vi "change_imagingMode.vi"(8 "error in (no error)":errorcluster, 10 "imagingModes":T1[](array[typedef]), 11 "imagingMode":refnum<vi>) -> (0 "error out":errorcluster)   [LabVIEW 2010]
uses:
  common/clusters/plugin_specification.ctl
  components/ImagingMode/GenericImagingMode/GenericImagingMode/GenericImagingMode.lvclass
  common/classes/GenericComponent/GenericComponent/GenericComponent.lvclass
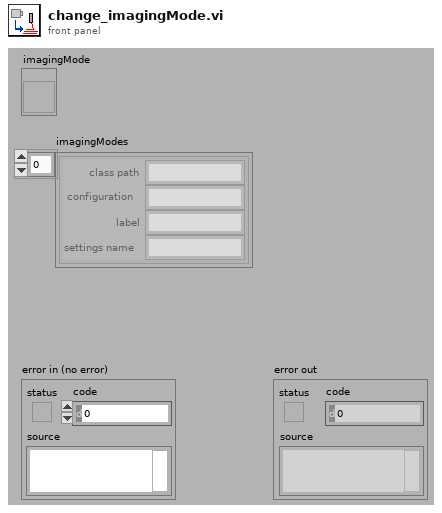
[diagram p1: front panel]
types:
  T1 = typedef "plugin_specification.ctl" = cluster{"class path":string, "configuration":string, "label":string, "settings name":string}
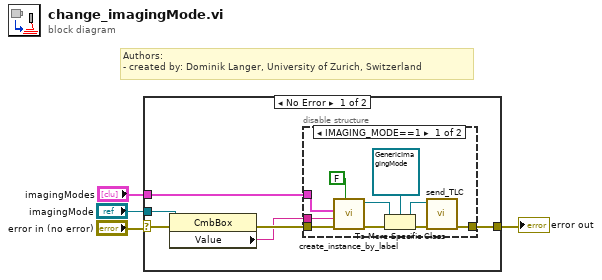
[diagram p0: block diagram]
diagram:
  # "Authors: \n- created by: Dominik Langer, University of Zurich, Switzerland"
  n1 = case shown="No Error" "error in (no error)" {
    selector: "error in (no error)" -> [w9 w22]
    tunnel: [w10 w22] -> w4
    tunnel: "imagingMode" -> [w6 _]
    tunnel: "imagingModes" -> [w5 _]
    frame No Error {
      n2 = property class="CmbBox"(reference=w6, error in=w9) -> (error out=w8:errorcluster, "Value"=w7:string)  [unwired: 1 out]
      n3 = disable-structure shown="IMAGING_MODE==1" {
        disable-tunnel: w8 -> [w16 w21]
        disable-tunnel: [w19 w21] -> w10
        disable-tunnel: w7 -> [w12 _]
        disable-tunnel: w5 -> [w11 _]
        frame condition #0 (active) {
          n4 = call "create_instance_by_label.vi"("call constructor?"=FALSE, "error in (no error)"=w16, "label"=w12, "configuration list"=w11) -> ("error out"=w15:errorcluster, "GenericPlugin out"=w14:refnum<class "GenericComponent.lvclass">)  [unwired: 6 out]
          n5 = To More Specific Class(target class=refnum<class "GenericImagingMode.lvclass"> refnum ("GenericScanMode.lvclass"), reference=w14, error in=w15) -> (specific class reference=w18:refnum<class "GenericImagingMode.lvclass">, error out=w17:errorcluster)
          n6 = call-dynamic "send_TLC.vi"("error in (no error)"=w17, "GenericScanMode in"=w18) -> ("error out"=w19:errorcluster)  [unwired: 8 in, 1 out]
        }
        frame condition #1 {
        }
      }
    }
    frame Error {
    }
  }
  "error out" <- w4
